vi "2014 Ball Detection.vi"() -> ()   [LabVIEW 2013]
uses:
  <vilib>/Rock Robotics/WPI/Camera/WPI_CameraSettings Read MJPG.ctl
  <vilib>/Rock Robotics/WPI/Camera/WPI_CameraImageSize.ctl
  <vilib>/ptbypt/NI_PtbyPt.lvlib
panel:
  in  "Path":path
  out "distance from center":sgl
  out "distance":dbl
  out "Object Info[0].Fitted Circle.Radius (Pixels)":dbl
  in  "Std Devs":cluster{"Hue":dbl, "Sat":dbl, "Val":dbl}={"Hue"=4.0, "Sat"=6.0, "Val"=4.0}
  in  "Targets":i32=3
  in  "Area Size Limit %":dbl=0.4 format="%#_13g"
  in  "Instructions:":string="Use the tab immediately below to choose the image source. Update the camera settings or the image directory so that you have images or video to test with.\n\nCalibration:\nYou can update Color Component ranges directly, or by clicking and drawing a line across the upper third of a ball within the image -- example shown below-right.\n\nUse Debugging tab to view intermediate results. Adjust Std Dev multipliers and line to achieve the desired HSV upper and lower threshold limits.\n\nArea Size LImit is used to ignore objects too small or balls too far away to care about.\n\nTargets identifies how many of the top scores to return.\n\nThe Details tab contains center, radius, and score details of each object."
  out "loop time ms":u32
  in  "Score Cutoff":dbl(slide)=70.58823529411765 scale=0.0..100.0
  in  "Color Components":T1={"Hue"={243.23333311080933, 20.233333110809326}, "Sat"={125.60287475585938, 242.93045043945312}, "Val"={83.88507843017578, 225.38158416748047}} {"Val" scale=0.0..255.0; "Sat" scale=0.0..255.0; "Hue" scale=0.0..255.0 scale format="%#_3g"}
  out "Error":bool
  in  "Image Source":enum32{"Files", "Camera"}(tab)
  in  "List of image files":i32(listbox)
  in  "Image Directory":path=path "2014 Vision Target"
  in  "Camera Settings":T2={"fps"=15, "compression"=5, "Image Size"=enum."320x240"}
  in  "Camera IP":string="10.04.19.11"
  in  "Tabbed Info":enum32{"Debugging", "Details"}(tab)
  in  "Annotations":enum16{"None", "Good", "All"}(ring)=enum."Good"
  out "Initial Mask":T4(plugin-control)
  out "Fitted Mask":T4(plugin-control)
  out "Ranked Objects":T5(array[cluster]) {"Score" format="%#.1g"}
  out "Image":T4(plugin-control)
  # "Ranking Colors:\n1. green\n2. cyan\n3. magenta\n4. orange"
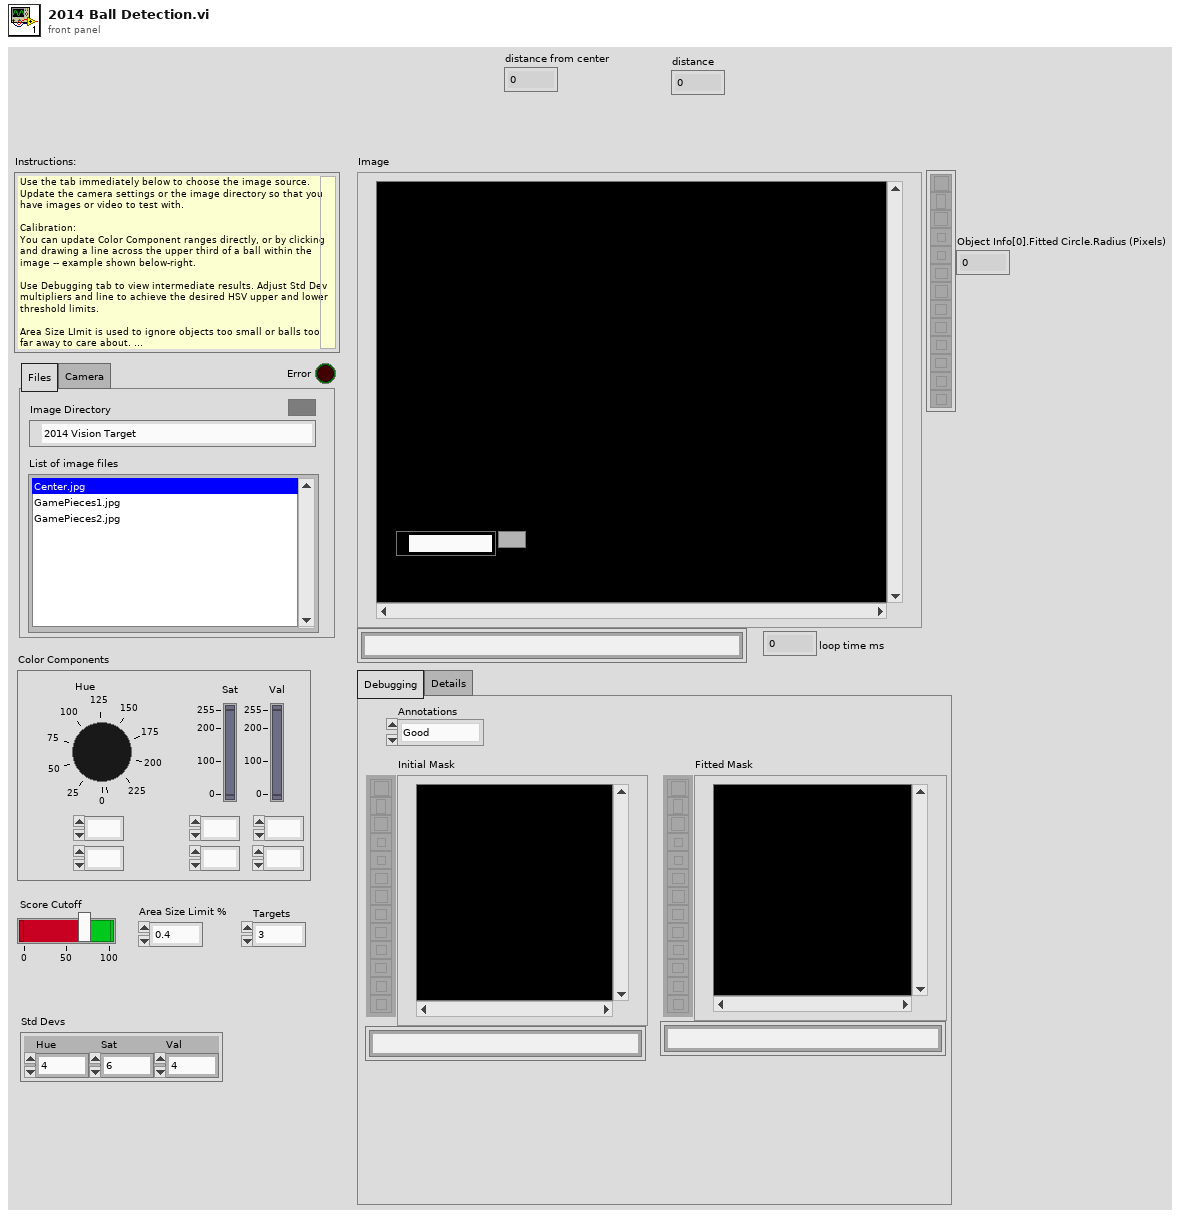
[diagram p1: front panel]
types:
  T1 = cluster{"Hue":cluster{dbl, dbl}, "Sat":cluster{dbl, dbl}, "Val":cluster{dbl, dbl}}
  T2 = typedef "WPI_CameraSettings Read MJPG.ctl" = cluster{"fps":i32, "compression":i32, "Image Size":T3}
  T3 = typedef "WPI_CameraImageSize.ctl" = enum16{"640x480", "320x240", "160x120"}
  T4 = typedef "IMAQ Image.ctl" = refnum<image>
  T5 = cluster{"Score":sgl, "Fitted Circle":cluster{"Center":cluster{"X":sgl, "Y":sgl}, "Radius":dbl, "Circle Rect":cluster{"L":sgl, "T":sgl, "R":sgl, "B":sgl}, "Roundness":dbl, "SNR (dB)":dbl}, "Search Rect":cluster{"L":sgl, "T":sgl, "R":sgl, "B":sgl}, "Details":cluster{"Edge":sgl, "Area":sgl, "Circ":sgl, "Diam":sgl}}[]
  T6 = typedef "Image Type" = u32
  T7 = cluster{"Circle Found":bool, "Fitted Circle":cluster{"Center":cluster{"X":sgl, "Y":sgl}, "Radius":dbl, "Center":cluster{"X":sgl, "Y":sgl}, "Radius":dbl, "Roundness":dbl, "Strength":dbl, "SNR (dB)":dbl}, "Array":dbl[], "Sorted Data":dbl[][]}[]
  T8 = cluster{cluster{dbl, dbl}, cluster{dbl, dbl}, cluster{dbl, dbl}}
  T9 = cluster{"Score":dbl, "Fitted Circle":cluster{"Center (Pixels)":cluster{"X":sgl, "Y":sgl}, "Radius (Pixels)":dbl, "Circle Rect":cluster{"Left":sgl, "Top":sgl, "Right":sgl, "Bottom":sgl}, "Roundness (RW)":dbl, "Average SNR (dB)":dbl}, "Search Rect":cluster{"Left":sgl, "Top":sgl, "Right":sgl, "Bottom":sgl}, "Details":cluster{"Edges":sgl, "Circ/Rect":sgl, "Diam/Diam":sgl, "Circularity":sgl}}[]
  T10 = cluster{"Object Info[0]":cluster{"Score":dbl, "Fitted Circle":cluster{"Center (Pixels)":cluster{"X":sgl, "Y":sgl}, "Radius (Pixels)":dbl, "Circle Rect":cluster{"Left":sgl, "Top":sgl, "Right":sgl, "Bottom":sgl}, "Roundness (RW)":dbl, "Average SNR (dB)":dbl}, "Search Rect":cluster{"Left":sgl, "Top":sgl, "Right":sgl, "Bottom":sgl}, "Details":cluster{"Edges":sgl, "Circ/Rect":sgl, "Diam/Diam":sgl, "Circularity":sgl}}, "Object Info[1]":cluster{"Score":dbl, "Fitted Circle":cluster{"Center (Pixels)":cluster{"X":sgl, "Y":sgl}, "Radius (Pixels)":dbl, "Circle Rect":cluster{"Left":sgl, "Top":sgl, "Right":sgl, "Bottom":sgl}, "Roundness (RW)":dbl, "Average SNR (dB)":dbl}, "Search Rect":cluster{"Left":sgl, "Top":sgl, "Right":sgl, "Bottom":sgl}, "Details":cluster{"Edges":sgl, "Circ/Rect":sgl, "Diam/Diam":sgl, "Circularity":sgl}}, "Object Info[2]":cluster{"Score":dbl, "Fitted Circle":cluster{"Center (Pixels)":cluster{"X":sgl, "Y":sgl}, "Radius (Pixels)":dbl, "Circle Rect":cluster{"Left":sgl, "Top":sgl, "Right":sgl, "Bottom":sgl}, "Roundness (RW)":dbl, "Average SNR (dB)":dbl}, "Search Rect":cluster{"Left":sgl, "Top":sgl, "Right":sgl, "Bottom":sgl}, "Details":cluster{"Edges":sgl, "Circ/Rect":sgl, "Diam/Diam":sgl, "Circularity":sgl}}, "Object Info[3]":cluster{"Score":dbl, "Fitted Circle":cluster{"Center (Pixels)":cluster{"X":sgl, "Y":sgl}, "Radius (Pixels)":dbl, "Circle Rect":cluster{"Left":sgl, "Top":sgl, "Right":sgl, "Bottom":sgl}, "Roundness (RW)":dbl, "Average SNR (dB)":dbl}, "Search Rect":cluster{"Left":sgl, "Top":sgl, "Right":sgl, "Bottom":sgl}, "Details":cluster{"Edges":sgl, "Circ/Rect":sgl, "Diam/Diam":sgl, "Circularity":sgl}}, "Object Info[4]":cluster{"Score":dbl, "Fitted Circle":cluster{"Center (Pixels)":cluster{"X":sgl, "Y":sgl}, "Radius (Pixels)":dbl, "Circle Rect":cluster{"Left":sgl, "Top":sgl, "Right":sgl, "Bottom":sgl}, "Roundness (RW)":dbl, "Average SNR (dB)":dbl}, "Search Rect":cluster{"Left":sgl, "Top":sgl, "Right":sgl, "Bottom":sgl}, "Details":cluster{"Edges":sgl, "Circ/Rect":sgl, "Diam/Diam":sgl, "Circularity":sgl}}, "Object Info[5]":cluster{"Score":dbl, "Fitted Circle":cluster{"Center (Pixels)":cluster{"X":sgl, "Y":sgl}, "Radius (Pixels)":dbl, "Circle Rect":cluster{"Left":sgl, "Top":sgl, "Right":sgl, "Bottom":sgl}, "Roundness (RW)":dbl, "Average SNR (dB)":dbl}, "Search Rect":cluster{"Left":sgl, "Top":sgl, "Right":sgl, "Bottom":sgl}, "Details":cluster{"Edges":sgl, "Circ/Rect":sgl, "Diam/Diam":sgl, "Circularity":sgl}}, "Object Info[6]":cluster{"Score":dbl, "Fitted Circle":cluster{"Center (Pixels)":cluster{"X":sgl, "Y":sgl}, "Radius (Pixels)":dbl, "Circle Rect":cluster{"Left":sgl, "Top":sgl, "Right":sgl, "Bottom":sgl}, "Roundness (RW)":dbl, "Average SNR (dB)":dbl}, "Search Rect":cluster{"Left":sgl, "Top":sgl, "Right":sgl, "Bottom":sgl}, "Details":cluster{"Edges":sgl, "Circ/Rect":sgl, "Diam/Diam":sgl, "Circularity":sgl}}, "Object Info[7]":cluster{"Score":dbl, "Fitted Circle":cluster{"Center (Pixels)":cluster{"X":sgl, "Y":sgl}, "Radius (Pixels)":dbl, "Circle Rect":cluster{"Left":sgl, "Top":sgl, "Right":sgl, "Bottom":sgl}, "Roundness (RW)":dbl, "Average SNR (dB)":dbl}, "Search Rect":cluster{"Left":sgl, "Top":sgl, "Right":sgl, "Bottom":sgl}, "Details":cluster{"Edges":sgl, "Circ/Rect":sgl, "Diam/Diam":sgl, "Circularity":sgl}}, "Object Info[8]":cluster{"Score":dbl, "Fitted Circle":cluster{"Center (Pixels)":cluster{"X":sgl, "Y":sgl}, "Radius (Pixels)":dbl, "Circle Rect":cluster{"Left":sgl, "Top":sgl, "Right":sgl, "Bottom":sgl}, "Roundness (RW)":dbl, "Average SNR (dB)":dbl}, "Search Rect":cluster{"Left":sgl, "Top":sgl, "Right":sgl, "Bottom":sgl}, "Details":cluster{"Edges":sgl, "Circ/Rect":sgl, "Diam/Diam":sgl, "Circularity":sgl}}}
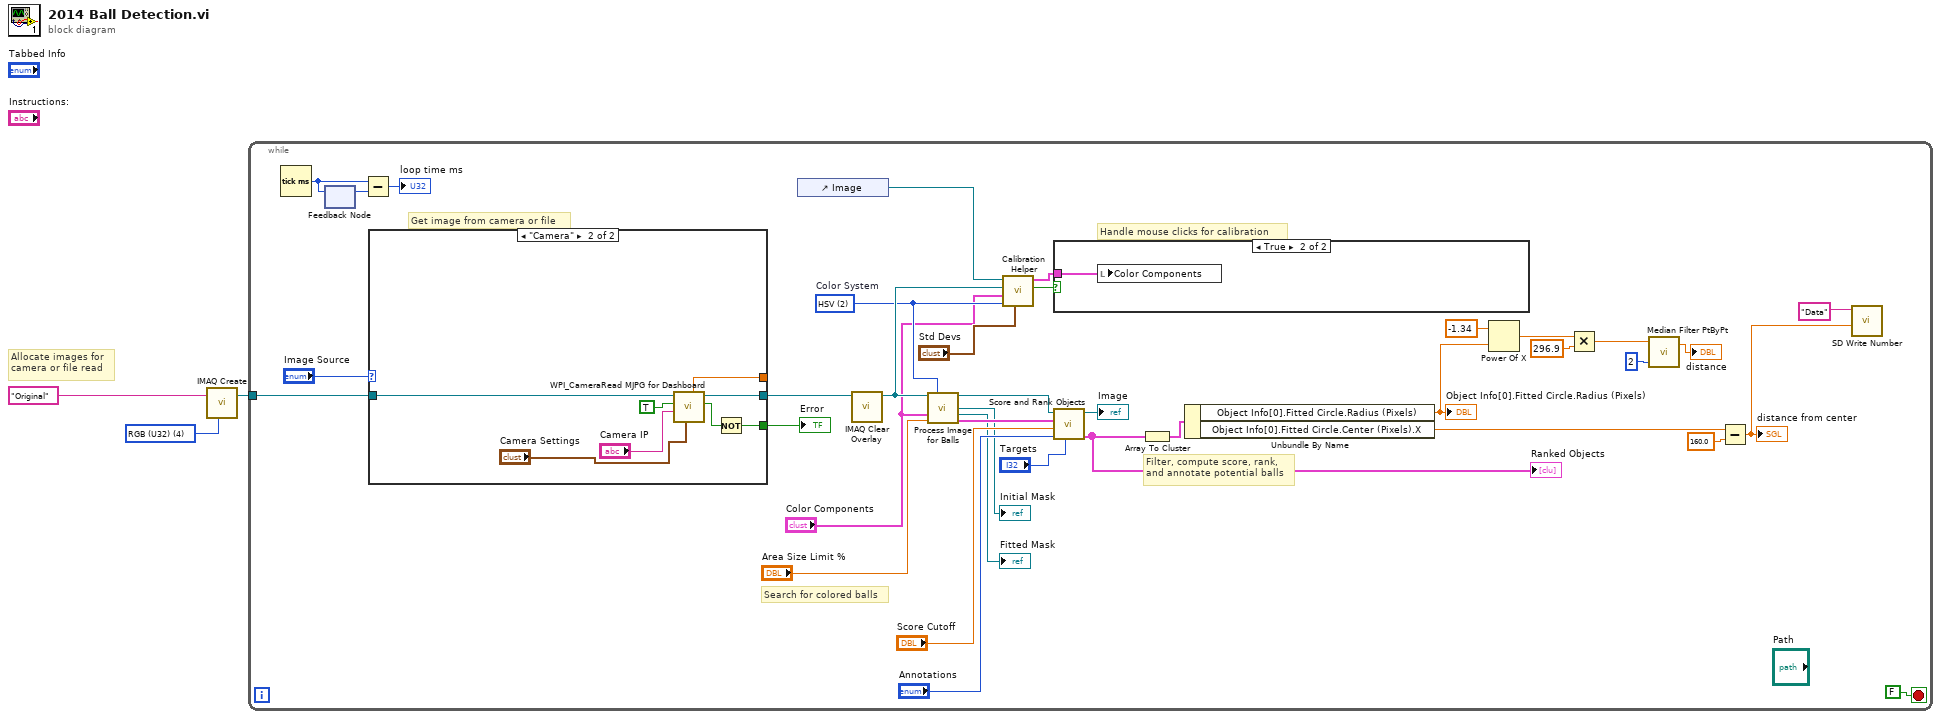
[diagram p0: block diagram]
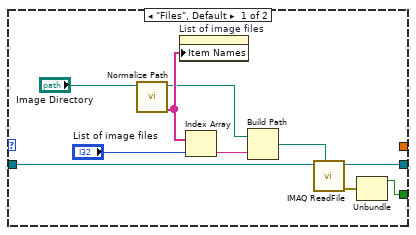
[diagram p3: hidden frame]
diagram:
  w3 = T6 4 items=["Grayscale (U8)", "Grayscale (I16)", "Grayscale (SGL)", "Complex (CSG)", "RGB (U32)", "HSL (U32)", "RGB (U64)", "Grayscale (U16)"] ("Image Type")
  # "Allocate images for\ncamera or file read"
  n1 = call "IMAQ Create"("Image Name"="Original", "Image Type"=w3) -> ("New Image"=w1:T4)  [unwired: 3 in, 1 out]
  n2 = while {
    tunnel: w1 -> [w37]
    stop <- FALSE stop-if-true
    w22 = u16 2 items=["RGB", "HSL", "HSV", "HSI"]  # Color System
    # "Handle mouse clicks for calibration"
    # "Search for colored balls"
    # "Filter, compute score, rank,\nand annotate potential balls"
    # "Get image from camera or file"
    n3 = Tick Count (ms)() -> (millisecond timer value=w35:u32)
    n4 = feedback #1() -> (w34:u32)  [unwired: 1 in]
    n5 = feedback-in #1(w35) -> ()
    n6 = Subtract(x=w35, y=w34) -> (x-y=→"loop time ms":u32)
    n7 = case shown="\"Camera\"" "Image Source" {
      tunnel: [w48 w58] -> w40
      tunnel: w37 -> [w47 w59]
      tunnel: [w45 w53] -> w36
      tunnel: [_ w52] -> _
      frame "Files", Default {
        n8 = call "Normalize Path.vi"("Image Directory"="Image Directory") -> ("Filenames"=w44:string[], "Path"=w42:path)  [unwired: 9 in]
        n9 = property on="List of image files" class="LstBox (strict)"("Item Names"=w44) -> ()  [unwired: 2 in, 2 out]
        n10 = Index Array(array=w44, index="List of image files") -> (element=w50:string)
        n11 = Build Path(base path=w42, name or relative path=w50) -> (appended path=w49:path)
        n12 = call "IMAQ ReadFile"("File Path"=w49, "Image"=w47) -> ("error out"=w46:errorcluster, "Image Out"=w48:T4)  [unwired: 5 in, 3 out]
        n13 = Unbundle(w46) -> ("status"=w45:bool)  [unwired: 2 out]
      }
      frame "Camera" {
        n14 = call <vilib>:"WPI_CameraRead MJPG for Dashboard.vi"("Camera Settings"="Camera Settings", "Camera IP"="Camera IP", "Enable"=TRUE, "Refnum in"=w59) -> ("Active"=w55:bool, "Refnum out"=w58:T4, "Bandwidth (Mbps)"=w52:dbl)  [unwired: 4 in, 1 out]
        n15 = Not(x=w55) -> (.not. x?=w53:bool)
      }
    }
    "Error" <- w36
    n16 = control-ref of="Image"() -> (w21:refnum<vi>)
    n17 = call "IMAQ Clear Overlay"("Image"=w40) -> ("Image Out"=w29:T4)  [unwired: 9 in, 1 out]
    n18 = call "Process Image for Balls.vi"("Src Image"=w29, "Color Mode 2"=w22, "Color"="Color Components", "Area Cutoff %"="Area Size Limit %") -> ("Src Image Out"=w27:T4, "First Threshold"=→"Initial Mask":T4, "Fitted"=→"Fitted Mask":T4, "Potential"=w26:T7)  [unwired: 8 in]
    n19 = call "Calibration Helper.vi"("Std Devs"="Std Devs", "Color Mode"=w22, "Color Components"="Color Components", "Image"=w29, "Image Ctl Refnum"=w21) -> ("Changed"=w18:bool, "output color"=w20:T8)  [unwired: 5 in]
    n20 = case shown="True" w18 {
      tunnel: w20 -> [_ w41]
      frame False {
      }
      frame True {
        n21 = local write "Color Components"(w41) -> ()
      }
    }
    n22 = call "Score and Rank Objects.vi"("Targets"="Targets", "Annotations"="Annotations", "Score Limit"="Score Cutoff", "Object Info"=w26, "Image in"=w27) -> ("Object Info"=w16:T9, "Annotated Image"=→"Image":T4)  [unwired: 5 in]
    "Ranked Objects" <- w16
    n23 = Array To Cluster(array=w16) -> (cluster=w15:T10)
    n24 = Unbundle By Name(w15) -> ("Object Info[0].Fitted Circle.Radius (Pixels)"=w11:dbl, "Object Info[0].Fitted Circle.Center (Pixels).X"=w8:sgl)
    "Object Info[0].Fitted Circle.Radius (Pixels)" <- w11
    n25 = Power Of X(1:w11, 2:-1.34 ("y")) -> (0:w13:dbl)
    n26 = Multiply(x=w13, y=296.9) -> (x*y=w9:dbl)
    n27 = call <vilib>:"Median Filter PtByPt.vi"("rank"=2, "x"=w9) -> ("Filtered x"=→"distance":dbl)  [unwired: 2 in, 1 out]
    n28 = Subtract(x=w8, y=sgl 160.0) -> (x-y=w4:sgl)
    "distance from center" <- w4
    n29 = call <vilib>:"SD Write Number.vi"("Numeric"=w4, "Name"="Data") -> ()  [unwired: 8 in, 2 out]
  }
